vi "Send Voltage.vi"(8 "error in (no error)":errorcluster, 11 "57XX in":refnum<class "57XX.lvclass">) -> (0 "error out":errorcluster, 3 "57XX out":refnum<class "57XX.lvclass">)   [LabVIEW 2019, in "57XX.lvlib" / "57XX.lvclass"]
uses:
  Library/57XX.lvclass
  C:/Users/Public/Documents/Development/builds/Instruments/PowerSupply.lvlibp/Library/PowerSupply.lvclass
  Library/57XX.lvclass/57XX.ctl
  Accessors/Read Local Resource.vi
  Accessors/Write Local Resource.vi
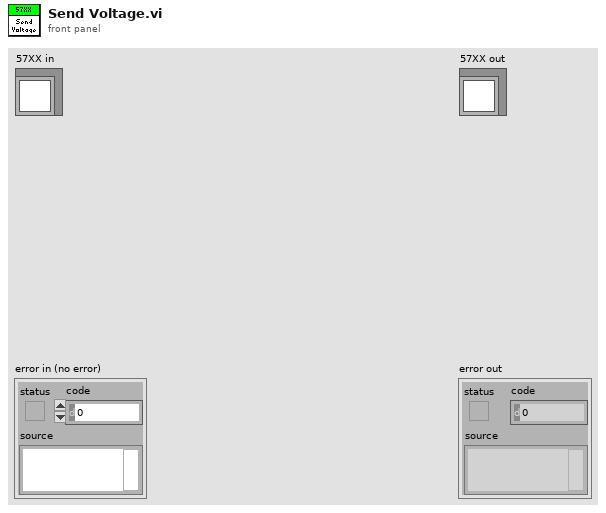
[diagram p1: front panel]
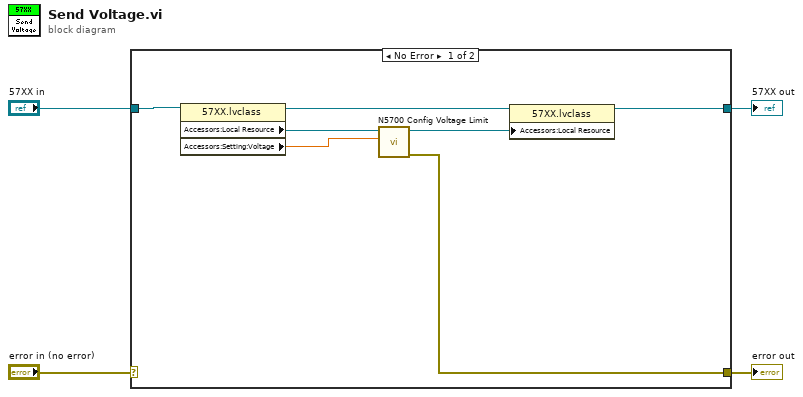
[diagram p0: block diagram]
diagram:
  n1 = case shown="No Error" "error in (no error)" {
    selector: "error in (no error)" -> [_ w13]
    tunnel: [w8 w13] -> w3
    tunnel: [w5 w12] -> w1
    tunnel: "57XX in" -> [w11 w12]
    frame No Error {
      n2 = property class="57XX.lvclass"(reference=w11) -> (reference out=w6:refnum<class "57XX.lvclass">, "Accessors:Local Resource"=w10:refnum<visa-resource-name>, "Accessors:Setting:Voltage"=w9:dbl)  [unwired: 1 in, 1 out]
      n3 = call <instrlib>:"N5700 Config Voltage Limit.vi"("Volt Limit"=w9, "VISA"=w10) -> ("error out"=w8:errorcluster, "VISA out"=w7:refnum<visa-resource-name>)  [unwired: 5 in]
      n4 = property class="57XX.lvclass"(reference=w6, "Accessors:Local Resource"=w7) -> (reference out=w5:refnum<class "57XX.lvclass">)  [unwired: 1 in, 1 out]
    }
    frame Error {
    }
  }
  "error out" <- w3
  "57XX out" <- w1
